vi "Types.vi"(8 "error in (no error)":errorcluster, 11 "Control List in":refnum<class "Control List.lvclass">) -> (0 "error out":errorcluster, 2 "Types":string[](array[string]), 3 "Control List out":refnum<class "Control List.lvclass">)   [LabVIEW 2020, in "VolatusGUIEditor.lvlib" / "Control List.lvclass"]
uses:
  Control List.lvclass
  Control List.lvclass/Control List.ctl
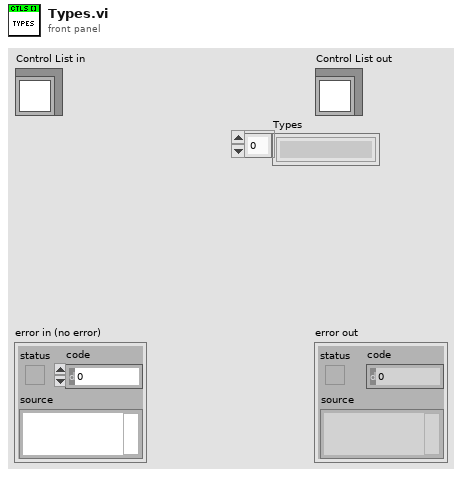
[diagram p1: front panel]
types:
  T1 = typedef "VolatusGUIEditor.lvlib/Control Info.ctl" = cluster{"Description":string, "Hierarchy":string[], "Image":T2, "Element Type":string, "Path":path}
  T2 = typedef "imagedata.ctl" = cluster{"image type":i32, "image depth":i32, "image":u8[], "mask":u8[], "colors":u32[], "Rectangle":cluster{"left":i16, "top":i16, "right":i16, "bottom":i16}}
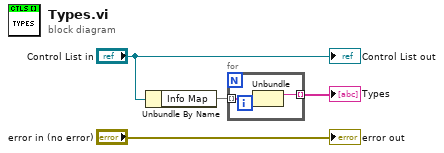
[diagram p0: block diagram]
diagram:
  n1 = Unbundle By Name("Control List in") -> ("Info Map"=w2:map{string, T1})
  n2 = for {
    tunnel: w2 -> [w6] mode=indexing
    tunnel: [w5] -> w1 mode=indexing
    n3 = Unbundle(w6) -> ("Control Type"=w5:string)  [unwired: 1 out]
  }
  "Types" <- w1
  "error out" <- "error in (no error)"
  "Control List out" <- "Control List in"
